vi "Initialize Configuration Display.vi"(8 "error in (no error)":errorcluster, 10 "Configuration Pane References":T1, 11 "Configuration in":refnum<class "Configuration.lvclass">) -> (0 "error out":errorcluster, 1 "Stop Event Loop":refnum<user-event>, 2 "Change Display":refnum<user-event>, 3 "Configuration out":refnum<class "Configuration.lvclass">)   [LabVIEW 2020, in "Configuration.lvlib" / "Configuration.lvclass"]
uses:
  Configuration.lvclass
  C:/Program Files/National Instruments/LabVIEW 2020/vi.lib/ActorFramework/Actor/Actor.lvclass
  Config Actor Core UI Ref.ctl
  <vilib>/ActorFramework/Actor/Actor.lvclass/Actor.ctl
  <vilib>/ActorFramework/Message Enqueuer/Message Enqueuer.lvclass/Message Enqueuer.ctl
  Configuration.lvclass/Configuration.ctl
  Configuration Messages/Display New Configuration SubPanel Msg/Display New Configuration SubPanel Msg.lvclass/Display New Configuration SubPanel Msg.ctl
  <vilib>/ActorFramework/Message Enqueuer/Init from Existing Queue.vi
  <vilib>/ActorFramework/Message Enqueuer/Enqueue.vi
  Configuration Messages/Display New Configuration SubPanel Msg/Display New Configuration SubPanel Msg.lvclass
  C:/Program Files/National Instruments/LabVIEW 2020/vi.lib/ActorFramework/Message/Message.lvclass
  <vilib>/ActorFramework/Message Priority Queue/Priority Enqueue.vi
  <vilib>/ActorFramework/Message Enqueuer/Message Enqueuer.lvclass
  <vilib>/ActorFramework/Actor/Actor.lvclass
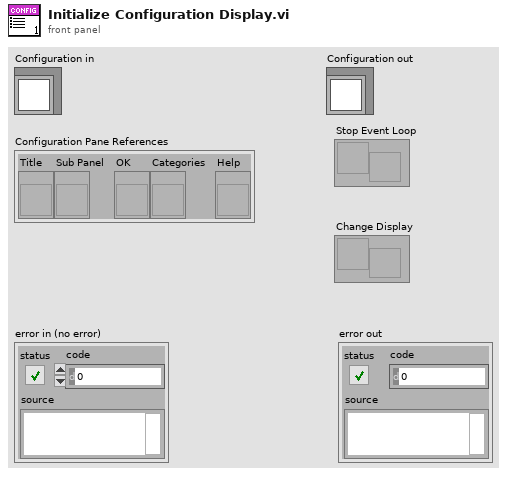
[diagram p1: front panel]
types:
  T1 = typedef "Configuration.lvlib/Configuration.lvclass/Config Actor Core UI Ref.ctl" = cluster{"Title":refnum<vi>, "Sub Panel":refnum<vi>, "OK":refnum<vi>, "Categories":refnum<vi>, "Help":refnum<vi>}
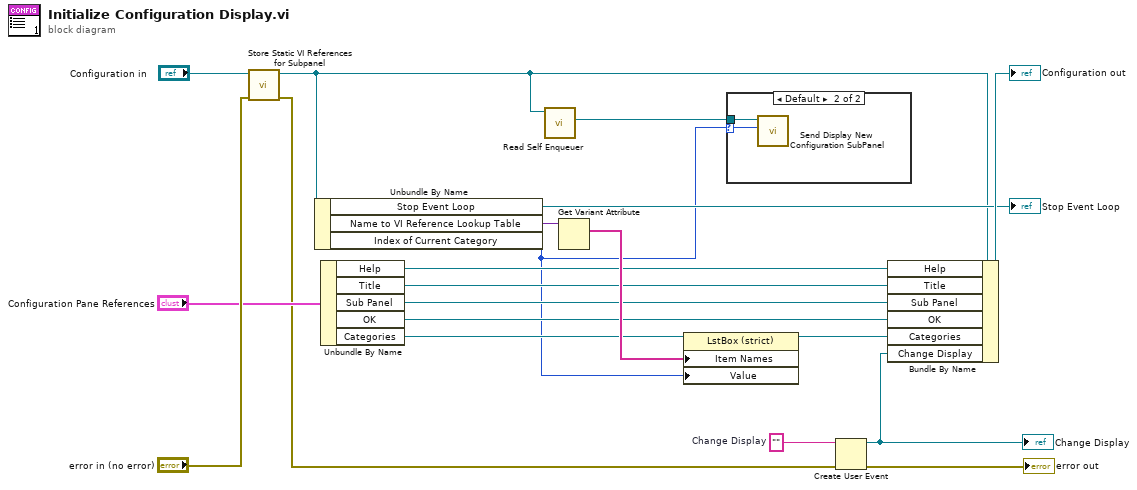
[diagram p0: block diagram]
diagram:
  w19 = ""  # Change Display
  n1 = call-dynamic "Store Static VI References for Subpanel.vi"("error in (no error)"="error in (no error)", "Configuration in"="Configuration in") -> ("error out"=w2:errorcluster, "Configuration out"=w4:refnum<class "Configuration.lvclass">)  [unwired: 8 in]
  n2 = Unbundle By Name(w4) -> ("Stop Event Loop"=→"Stop Event Loop":refnum<user-event>, "Name to VI Reference Lookup Table"=w15:variant, "Index of Current Category"=w1:i32)
  n3 = Unbundle By Name("Configuration Pane References") -> ("Help"=w5:refnum<vi>, "Title"=w10:refnum<vi>, "Sub Panel"=w9:refnum<vi>, "OK"=w8:refnum<vi>, "Categories"=w7:refnum<vi>)
  n4 = call <vilib>:"Read Self Enqueuer.vi"("Actor"=w4) -> ("Self Enqueuer"=w3:refnum<class "Message Enqueuer.lvclass">)  [unwired: 10 in]
  n5 = Get Variant Attribute(Variant=w15) -> (names=w14:string[])  [unwired: 3 in, 3 out]
  n6 = property class="LstBox (strict)"(reference=w7, "Item Names"=w14, "Value"=w1) -> (reference out=w12:refnum<vi>)  [unwired: 1 in, 1 out]
  n7 = case shown="Default" w1 {
    selector: w1 -> [_ w21]
    tunnel: w3 -> [_ w22]
    frame -1 {
    }
    frame Default {
      n8 = call "Send Display New Configuration SubPanel.vi"("ListBox Selection"=w21, "Message Enqueuer"=w22) -> ()  [unwired: 8 in, 2 out]
    }
  }
  n9 = Create User Event(user event datatype=w19, error in=w2) -> (user event=w20:refnum<user-event>, error out=→"error out":errorcluster)
  "Change Display" <- w20
  n10 = Bundle By Name(cluster=w4, "Help"=w5, "Title"=w10, "Sub Panel"=w9, "OK"=w8, "Categories"=w12, "Change Display"=w20) -> (→"Configuration out":refnum<class "Configuration.lvclass">)
